vi "Read from File.vi"(8 "error in (no error)":errorcluster, 10 "INI Ref":T1, 11 "Numeric Assertion in":refnum<class "Numeric Assertion.lvclass">) -> (0 "error out":errorcluster, 2 "INI Ref out":T1, 3 "Numeric Assertion out":refnum<class "Numeric Assertion.lvclass">)   [LabVIEW 2020, in "MacroAssert.lvlib" / "Numeric Assertion.lvclass"]
uses:
  Numeric Assertion.lvclass
  C:/Users/acasalen/Documents/LabVIEW Data/Projects/MacroAssert/source/Classes/Step/Step.lvclass
  <vilib>/Utility/config.llb/Config Data RefNum.ctl
  <vilib>/Utility/config.llb/Read Key (String).vi
  Assertion Step/Assertion Step.lvclass
  <vilib>/Utility/config.llb/NI_LVConfig.lvlib
  MacroAssert.lvlib
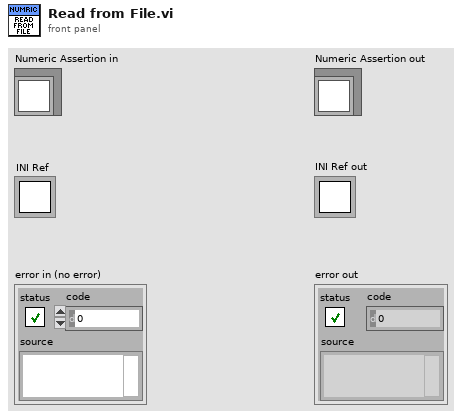
[diagram p1: front panel]
types:
  T1 = typedef "NI_LVConfig.lvlib/Config Data RefNum.ctl" = refnum<k1>
  T2 = enum8{"Enabled", "Disabled", "Disabled and Grayed Out"}
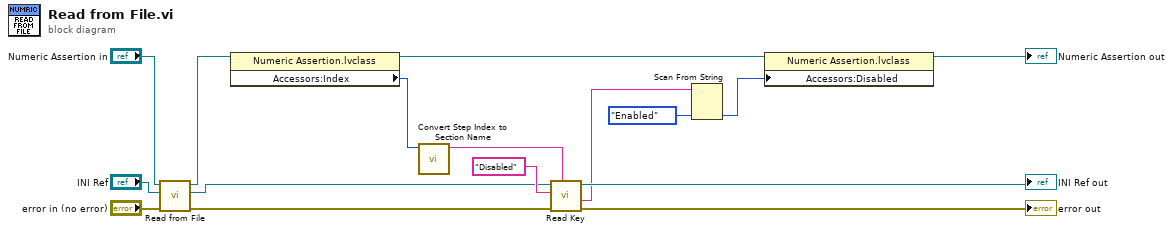
[diagram p0: block diagram]
diagram:
  n1 = call-parent "Read from File.vi"("error in (no error)"="error in (no error)", "INI Ref"="INI Ref", "Assertion Step in"="Numeric Assertion in") -> ("error out"=w9:errorcluster, "INI Ref out"=w4:T1, "Assertion Step out"=w8:refnum<class "Numeric Assertion.lvclass">)  [unwired: 6 in]
  n2 = property class="Numeric Assertion.lvclass"(reference=w8) -> (reference out=w12:refnum<class "Numeric Assertion.lvclass">, "Accessors:Index"=w11:i32)  [unwired: 1 in, 1 out]
  n3 = call "Convert Step Index to Section Name.vi"("Step Index"=w11) -> ("Section Name"=w10:string)  [unwired: 10 in]
  n4 = call-poly <vilib>:"Read Key.vi"("section"=w10, "error in (no error)"=w9, "key"="Disabled", "refnum"=w4) -> ("error out"=→"error out":errorcluster, "value"=w2:string, "refnum out"=→"INI Ref out":T1)  [unwired: 4 in, 1 out]
  n5 = Scan From String(input string=w2, default 1=T2."Enabled" ("Disabled")) -> (output 1=w1:T2)  [unwired: 3 in, 3 out]
  n6 = property class="Numeric Assertion.lvclass"(reference=w12, "Accessors:Disabled"=w1) -> (reference out=→"Numeric Assertion out":refnum<class "Numeric Assertion.lvclass">)  [unwired: 1 in, 1 out]
